vi "addBroadcastStepMotorFrame.vi"(8 "error in (no error)":errorcluster, 9 "TriggerIRQ":bool, 10 "WaitForTrigger":bool, 11 "Subnet in":refnum<class "Subnet.lvclass">) -> (0 "error out":errorcluster, 3 "Subnet out":refnum<class "Subnet.lvclass">)   [LabVIEW 2016, in "Subnet.lvclass"]
uses:
  Subnet.lvclass
  Subnet.lvclass/Subnet.ctl
  Common_RT_Modbus/IModbus/IModbus.lvclass
  Common_RT_HPILC/HPILC/HPILC.lvclass
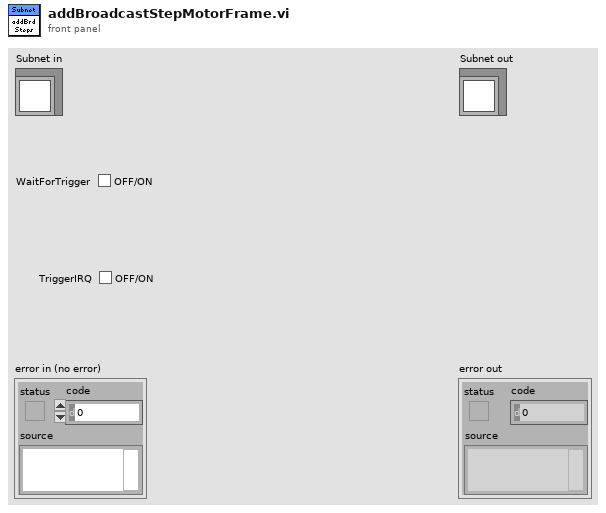
[diagram p1: front panel]
types:
  T1 = typedef "RTModbus.lvlib/TxFrame.ctl" = cluster{"Data":u8[], "WaitForTrigger":bool, "WaitForRx":u16, "TriggerIRQ":bool, "DelayMicroseconds":u16, "DelayMilliseconds":u16, "Timestamp":bool}
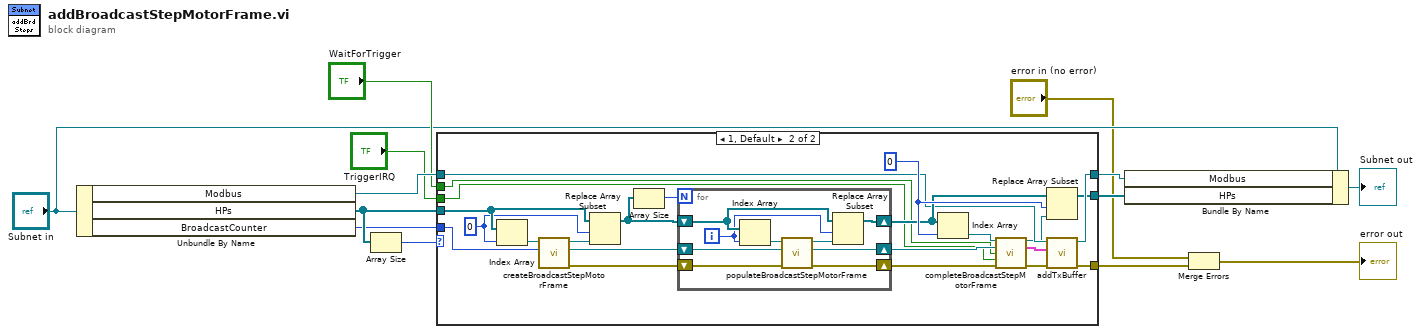
[diagram p0: block diagram]
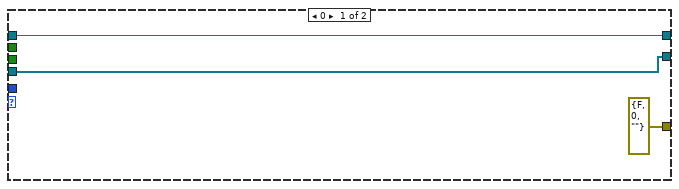
[diagram p2: hidden frame]
diagram:
  n1 = Unbundle By Name("Subnet in") -> ("Modbus"=w12:refnum<class "IModbus.lvclass">, "HPs"=w11:refnum<class "HPILC.lvclass">[], "BroadcastCounter"=w10:u8)
  n2 = Array Size(array=w11) -> (size(s)=w13:i32)
  n3 = case shown="1, Default" w13 {
    tunnel: w12 -> [w15 w24]
    tunnel: w11 -> [w16 w37]
    tunnel: w10 -> [_ w38]
    tunnel: "WaitForTrigger" -> [_ w27]
    tunnel: "TriggerIRQ" -> [_ w26]
    tunnel: [w15 w23] -> w5
    tunnel: [w16 w22] -> w4
    tunnel: [errorcluster {"status"=FALSE, "code"=0, "source"=""} ("error out") w18] -> w3
    frame 0 {
    }
    frame 1, Default {
      w31 = 0 ("index")
      w36 = 0 ("index")
      n4 = Index Array(array=w37, index=w36) -> (element=w39:refnum<class "HPILC.lvclass">)
      n5 = call "createBroadcastStepMotorFrame.vi"("BroadcastCounter"=w38, "HPILC in"=w39) -> ("error out"=w21:errorcluster, "FixedFrameBuilder"=w34:refnum<class "FixedFrameBuilder.lvclass">, "HPILC out"=w35:refnum<class "HPILC.lvclass">)  [unwired: 7 in]
      n6 = Replace Array Subset(array=w37, new element=w35, index=w36) -> (w33:refnum<class "HPILC.lvclass">[])
      n7 = Array Size(array=w33) -> (size(s)=w32:i32)
      n8 = for {
        N: w32 -> [_]
        shift-right: [w44] -> w28
        shift-left: w34 -> [w45]
        shift-right: [w42] -> w30
        shift-left: w33 -> [w48]
        shift-right: [w40] -> w20
        shift-left: w21 -> [w41]
        i -> [w47]
        n9 = Index Array(array=w48, index=w47) -> (element=w46:refnum<class "HPILC.lvclass">)
        n10 = call "populateBroadcastStepMotorFrame.vi"("error in (no error)"=w41, "FixedFrameBuilder in"=w45, "HPILC in"=w46) -> ("error out"=w40:errorcluster, "FixedFrameBuilder out"=w44:refnum<class "FixedFrameBuilder.lvclass">, "HPILC out"=w43:refnum<class "HPILC.lvclass">)  [unwired: 6 in]
        n11 = Replace Array Subset(array=w48, new element=w43, index=w47) -> (w42:refnum<class "HPILC.lvclass">[])
      }
      n12 = Index Array(array=w30, index=w31) -> (element=w29:refnum<class "HPILC.lvclass">)
      n13 = call "completeBroadcastStepMotorFrame.vi"("HPILC in"=w29, "FixedFrameBuilder"=w28, "WaitForTrigger"=w27, "TriggerIRQ"=w26, "error in (no error)"=w20) -> ("HPILC out"=w17:refnum<class "HPILC.lvclass">, "TxFrame"=w25:T1, "error out"=w19:errorcluster)  [unwired: 8 in]
      n14 = Replace Array Subset(array=w30, new element=w17, index=w31) -> (w22:refnum<class "HPILC.lvclass">[])
      n15 = call-dynamic "addTxBuffer.vi"("error in (no error)"=w19, "TxFrame"=w25, "IModbus in"=w24) -> ("error out"=w18:errorcluster, "IModbus out"=w23:refnum<class "IModbus.lvclass">)  [unwired: 7 in]
    }
  }
  n16 = Bundle By Name(cluster="Subnet in", "Modbus"=w5, "HPs"=w4) -> (→"Subnet out":refnum<class "Subnet.lvclass">)
  n17 = Merge Errors("error in (no error)", w3) -> (→"error out":errorcluster)
